vi "V50 Report Sample (SubVI).vi"(0 "NI_report in":refnum<class "NI_report.lvclass">, 5 "SampleID":string, 11 "error in (no error)":errorcluster) -> (4 "NI_report out":refnum<class "NI_report.lvclass">, 15 "error out":errorcluster)   [LabVIEW 2015]
uses:
  <vilib>/Utility/NIReport.llb/NI_report.lvclass
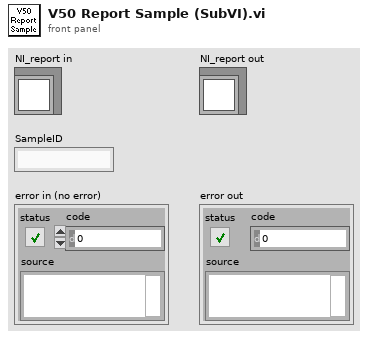
[diagram p1: front panel]
types:
  T1 = cluster{"position (excel)":cluster{"row":i32, "column":i32}, "name (excel)":string, "bookmark (word)":string}
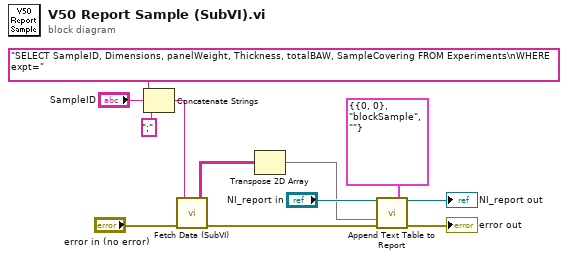
[diagram p0: block diagram]
diagram:
  n1 = Concatenate Strings("SELECT SampleID, Dimensions, panelWeight, Thickness, totalBAW, SampleCovering FROM Experiments\nWHERE expt=" ("query string"), "SampleID", ";" ("string")) -> (w9:string)
  n2 = call "Fetch Data (SubVI).vi"("error IN"="error in (no error)", "query string"=w9) -> ("error OUT"=w3:errorcluster, "recordset data"=w2:string[][])  [unwired: 4 out]
  n3 = Transpose 2D Array(2D array=w2) -> (transposed array=w1:string[][])
  n4 = call-dynamic "Append Text Table to Report.vi"("report in"="NI_report in", "MS Office parameters"=T1 {"position (excel)"={"row"=0, "column"=0}, "name (excel)"="blockSample", "bookmark (word)"=""}, "text data"=w1, "error in (no error)"=w3) -> ("report out"=→"NI_report out":refnum<class "NI_report.lvclass">, "error out"=→"error out":errorcluster)  [unwired: 8 in, 2 out]
